vi "小信号变比.vi"(6 "变比3":sgl, 8 "变比1":sgl, 9 "变比2":sgl, 11 "串口号":refnum<visa-resource-name>) -> (10 "应答":string)   [LabVIEW 2014]
panel:
  out "完整帧":u8[](array[numeric]) format="%.0x"
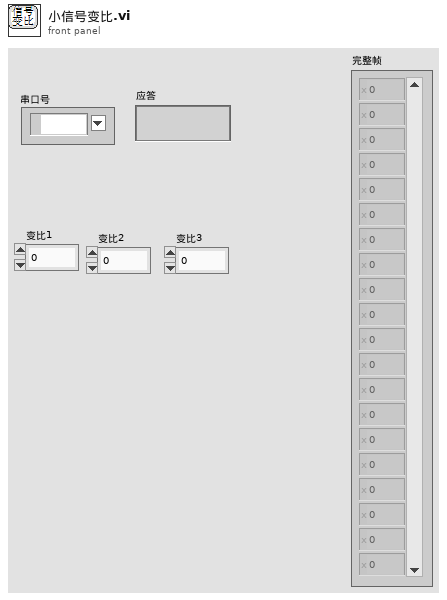
[diagram p1: front panel]
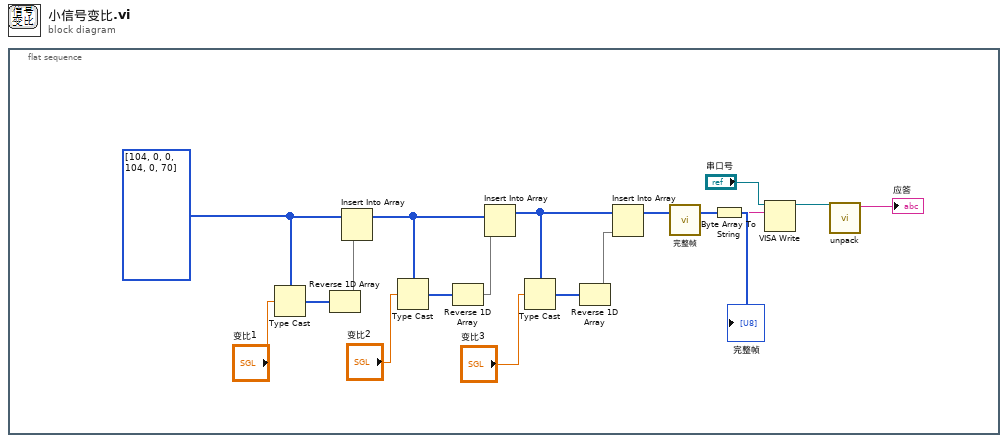
[diagram p0: block diagram]
diagram:
  n1 = flat-sequence {
    frame #0 {
      w10 = u8[] [104, 0, 0, 104, 0, 70]
      n2 = Type Cast(type=w10, x="变比1") -> (*(type *) &x=w12:u8[])
      n3 = Reverse 1D Array(array=w12) -> (reversed array=w9:u8[])
      n4 = Insert Into Array(array=w10, new element=w9) -> (w5:u8[])  [unwired: 1 in]
      n5 = Type Cast(type=w5, x="变比2") -> (*(type *) &x=w8:u8[])
      n6 = Reverse 1D Array(array=w8) -> (reversed array=w4:u8[])
      n7 = Insert Into Array(array=w5, new element=w4) -> (w3:u8[])  [unwired: 1 in]
      n8 = Type Cast(type=w3, x="变比3") -> (*(type *) &x=w7:u8[])
      n9 = Reverse 1D Array(array=w7) -> (reversed array=w2:u8[])
      n10 = Insert Into Array(array=w3, new element=w2) -> (w13:u8[])  [unwired: 1 in]
      n11 = call "完整帧.vi"("不完整帧"=w13) -> ("完整帧"=w18:u8[])  [unwired: 2 in]
      "完整帧" <- w18
      n12 = Byte Array To String(unsigned byte array=w18) -> (string=w17:string)
      n13 = VISA Write(VISA resource name="串口号", write buffer=w17) -> (VISA resource name out=w15:refnum<visa-resource-name>)  [unwired: 1 in, 2 out]
      n14 = call "unpack.vi"("串口号输入"=w15) -> ("应答"=→"应答":string)  [unwired: 5 in, 1 out]
    }
  }
